vi "rand_led_loop_test.vi"() -> ()   [LabVIEW 2012]
uses:
  <vilib>/Platform/TimedLoop/XDataNode/timing_clust.ctl
  <vilib>/Platform/TimedLoop/XDataNode/nitl_modes.ctl
  <vilib>/Platform/TimedLoop/XDataNode/wakeup.ctl
  <vilib>/rvi/Emulation/niFpgaSctlEmulationRegisterWithScheduler.vi
  <vilib>/rvi/Emulation/niFpgaSctlEmulationScheduler.vi
  <vilib>/Platform/TimedLoop/XDataNode/XDataNode.xnode
  <vilib>/Platform/TimedLoop/XDataNode/XDNodeRunTimeDep.lvlib
panel:
  out "Counter for receiving":u32
  out "Counter for sending":u32
  out "Sending test pulse?":bool
  out "Is Test Pulse?":bool
  out "Total number of pulses sent":u64
  in  "FPGA I/O In":refnum<k21>="IO Module\\D0 0"
  in  "Testpulse Time Delay (20 ns ticks)":u32=15
  in  "Testpulse duration (20 ns ticks)":u32=1
  in  "Testpulser On/Off":bool
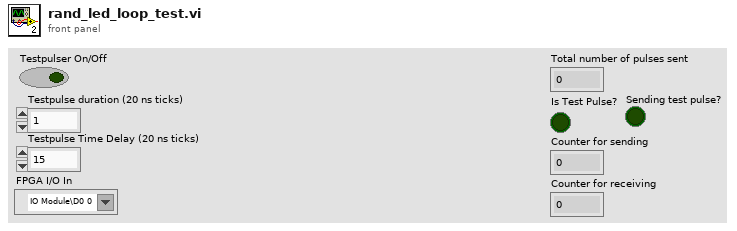
[diagram p1: front panel]
types:
  T1 = typedef "XDNodeRunTimeDep.lvlib/timing_clust.ctl" = cluster{"Expected End [f-1]":u64, "Actual End [f-1]":u64, "Finished Late? [f-1]":bool, "Expected End [i-1]":u64, "Actual End [i-1]":u64, "Finished Late? [i-1]":bool, "Expected Start [i]":u64, "Actual Start [i]":u64, "Expected Start [f]":u64, "Actual Start [f]":u64, "Source Name":string, "Structure Name":string, "Period":i64, "Deadline":i64, "Offset":i64, "Start":i64, "Priority":i32, "Timeout":i32, "Mode":T2, "Wakeup Reason":T3, "Error":errorcluster, "Source Type":string, "Secondary Source Type":string, "Global End Time":u64, "Global Start Time":u64, "Frame Duration":u64, "Iteration Duration":u64, "Assigned CPU":i32, "I/O Scan Engine Mode":u32}
  T2 = typedef "XDNodeRunTimeDep.lvlib/nitl_modes.ctl" = enum32{"No Change", "Process missed periods, maintain original phase", "Discard missed periods, maintain original phase", "Process missed periods, ignore original phase", "Discard missed periods, ignore original phase"}
  T3 = typedef "XDNodeRunTimeDep.lvlib/wakeup.ctl" = enum32{"Normal", "Aborted", "Asynchronous wakeup", "Timing source error", "Timed loop error", "Timeout"}
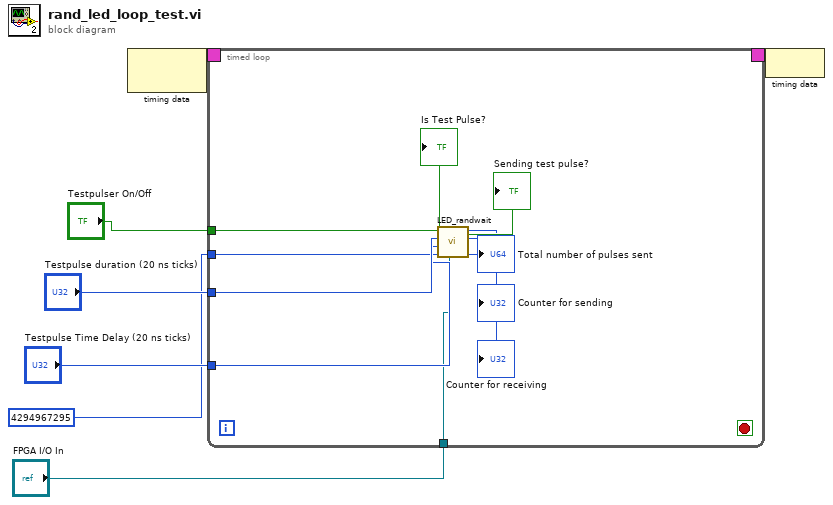
[diagram p0: block diagram]
diagram:
  n1 = node-c288() -> (w7:T1)  [unwired: 1 in]
  n2 = timed-loop {
    timing: w7 -> [_]
    timing-out: [_] -> w6
    tunnel: "Testpulser On/Off" -> [w17]
    tunnel: "Testpulse duration (20 ns ticks)" -> [w16]
    tunnel: "Testpulse Time Delay (20 ns ticks)" -> [w15]
    tunnel: u32 4294967295 ("seed") -> [w14]
    tunnel: "FPGA I/O In" -> [w13]
    stop <- _ stop-if-true
    n3 = call "LED_randwait.vi"("FPGA I/O In"=w13, "seed"=w14, "Testpulse Time Delay (20 ns ticks)"=w15, "Testpulse duration (20 ns ticks)"=w16, "Testpulser On/Off"=w17) -> ("Total number of pulses sent"=→"Total number of pulses sent":u64, "Counter for receiving"=→"Counter for receiving":u32, "Counter for sending"=→"Counter for sending":u32, "Sending test pulse?"=→"Sending test pulse?":bool, "Is Test Pulse?"=→"Is Test Pulse?":bool)  [unwired: 2 in]
  }
  n4 = node-c288(w6) -> ()
